vi "Pre-allocated.vi"(8 "error in (no error)":errorcluster, 11 "Test Data in":T1) -> (0 "error out":errorcluster, 3 "Test Data out":T1)   [LabVIEW 2024, in "Tester.lvlib"]
uses:
  Tester.lvlib
  test_data--cluster.ctl
  packetized_data--cluster.ctl
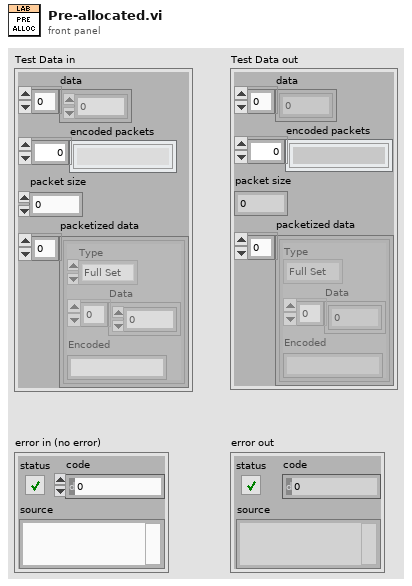
[diagram p1: front panel]
types:
  T1 = typedef "Tester.lvlib/test_data--cluster.ctl" = cluster{"data":dbl[], "encoded packets":string[], "packet size":i32, "packetized data":T2[]}
  T2 = typedef "Tester.lvlib/packetized_data--cluster.ctl" = cluster{"Type":enum16{"Full Set", "Last Set"}, "Data":dbl[], "Encoded":string}
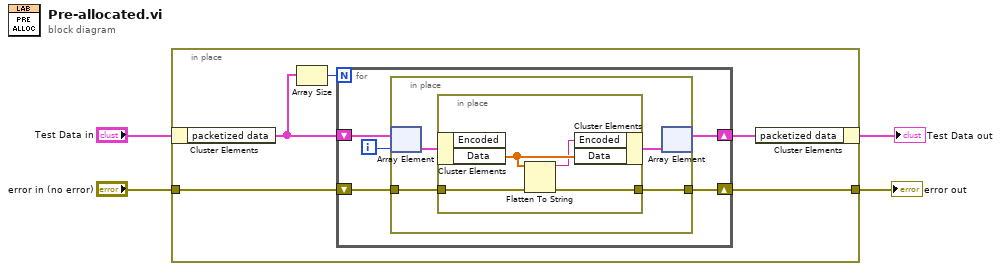
[diagram p0: block diagram]
diagram:
  n1 = in-place {
    in-place-border: "error in (no error)" -> [w6]
    in-place-border: [w5] -> w1
    n2 = in-place-cluster #1("Test Data in") -> ("packetized data"=w8:T2[])
    n3 = Array Size(array=w8) -> (size(s)=w9:i32)
    n4 = for {
      N: w9 -> [_]
      shift-right: [w13] -> w7
      shift-left: w8 -> [w14]
      shift-right: [w12] -> w5
      shift-left: w6 -> [w11]
      i -> [w10]
      n5 = in-place {
        in-place-border: [w17] -> w12
        in-place-border: w11 -> [w16]
        n6 = in-place-array #2(w14, w10) -> (w18:T2)
        n7 = in-place {
          in-place-border: [w21] -> w17
          in-place-border: w16 -> [w20]
          n8 = in-place-cluster #3(w18) -> ("Data"=w22:dbl[])  [unwired: 1 out]
          n9 = Flatten To String(anything=w22, error in (no error)=w20) -> (data string=w19:string, error out=w21:errorcluster)  [unwired: 2 in, 1 out]
          n10 = in-place-cluster #3("Encoded"=w19, "Data"=w22) -> (w15:T2)
        }
        n11 = in-place-array #2(w15) -> (w13:T2[])  [unwired: 1 out]
      }
    }
    n12 = in-place-cluster #1("packetized data"=w7) -> (→"Test Data out":T1)
  }
  "error out" <- w1
